vi "Main.vi"() -> ()   [LabVIEW 2018, in "TemplatePatternDemo.lvclass"]
uses:
  TemplatePatternDemo.lvclass
  ConsoleOut/Print Options.ctl
  Game Class/Game.lvclass
  Cricket Class/Cricket.lvclass
  C:/Users/fflores/Documents/LabVIEW-Open-Projects/LabIVEW OOP Design Patterns/Template Pattern/Game Class/Game.lvclass
  Football Class/Football.lvclass
panel:
  out "error out":errorcluster
  in  "Game Selector":enum16{"<Select a Game>", "Cricket", "Football"}(ring)
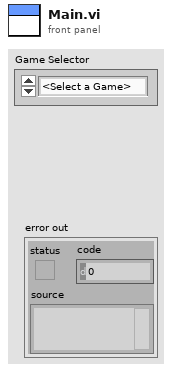
[diagram p1: front panel]
types:
  T1 = typedef "Print Options.ctl" = enum16{"Create", "Get Reference", "Print", "Print Header", "Close"}
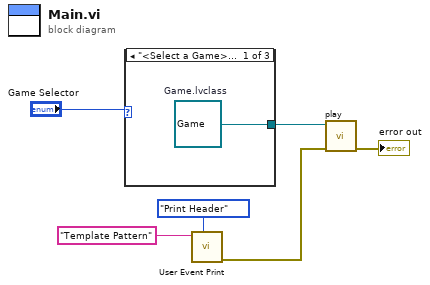
[diagram p0: block diagram]
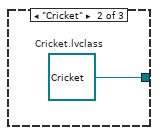
[diagram p2: hidden frame]
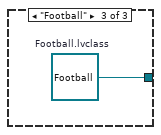
[diagram p3: hidden frame]
diagram:
  n1 = case shown="\"<Select a Game>\", Default" "Game Selector" {
    tunnel: [w7 w8 w9] -> w5
    frame "<Select a Game>", Default {
      w7 = refnum<class "Game.lvclass"> refnum  # Game.lvclass
    }
    frame "Cricket" {
      w8 = refnum<class "Cricket.lvclass"> refnum  # Cricket.lvclass
    }
    frame "Football" {
      w9 = refnum<class "Football.lvclass"> refnum  # Football.lvclass
    }
  }
  n2 = call "User Event Print.vi"("Options"=Print_Options."Print Header", "String to Print"="Template Pattern") -> ("error out"=w2:errorcluster)  [unwired: 8 in, 1 out]
  n3 = call "play.vi"("error in (no error)"=w2, "Game in"=w5) -> ("error out"=→"error out":errorcluster)  [unwired: 8 in, 1 out]
